vi "Normalize.vi"(8 "error in (no error)":errorcluster, 9 "Params":dbl[](array[numeric]), 10 "NISTData.NIDataArray":T3 {"Time Stamp" format="%^<%.3X\n%x>T"}, 11 "TVEMePe":dbl[][](array[numeric])) -> (0 "error out":errorcluster, 1 "Residual Histogram":T1(array[cluster]), 2 "MeanStdevSlopeSineAmpl":dbl[][](array[numeric]), 3 "Plot Out":cluster{dbl, "Time":dbl, dbl[][]}[](array[cluster]))   [LabVIEW 2014]
uses:
  typedefs/NIDataArray.ctl
  typedefs/NIData.ctl
  typedefs/PhasorRectangular.ctl
  <vilib>/Analysis/6fits.llb/Curve Fitting Criteria.ctl
  <vilib>/measure/matone.llb/Extract Single Tone Information 1 Chan.vi
  <vilib>/Analysis/NI_AALPro.lvlib
  <vilib>/Analysis/NI_AALBase.lvlib
  <vilib>/measure/NI_MAPro.lvlib
panel:
  out "Residual Error Distribution":T2(graph)
  out "Waveform Graph":cluster{dbl, "Time":dbl, dbl[][]}(graph)
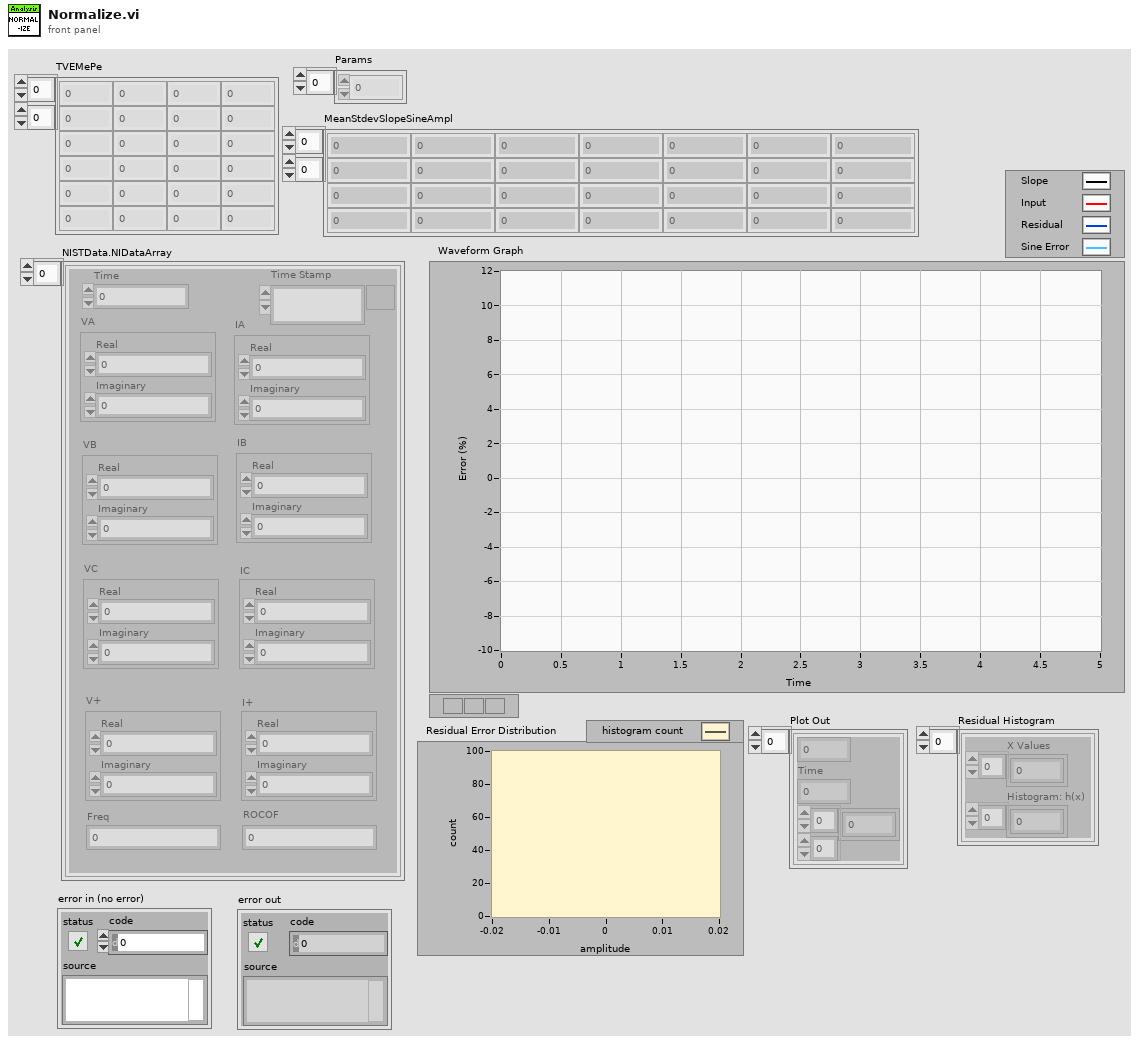
[diagram p1: front panel]
types:
  T1 = cluster{"X Values":dbl[], "Histogram: h(x)":i32[]}[]
  T2 = cluster{"X Values":dbl[], "Histogram: h(x)":i32[]}
  T3 = typedef "NIDataArray.ctl" = T4[]
  T4 = typedef "NIData.ctl" = cluster{"Time":dbl, "VA":T5, "VB":T5, "VC":T5, "V+":T5, "IA":T5, "IB":T5, "IC":T5, "I+":T5, "Freq":dbl, "ROCOF":dbl, "Time Stamp":timestamp}
  T5 = typedef "PhasorRectangular.ctl" = cluster{"Real":dbl, "Imaginary":dbl}
  T6 = enum32{"none", "input signal", "detected signal", "residual signal"}
  T7 = typedef "NI_AALPro.lvlib/Curve Fitting Criteria.ctl" = u16
  T8 = cluster{"exported time signal":waveform(dbl), "exported spectrum (dB)":cluster{"f0":dbl, "df":dbl, "dB Spectrum (Hann)":dbl[]}}
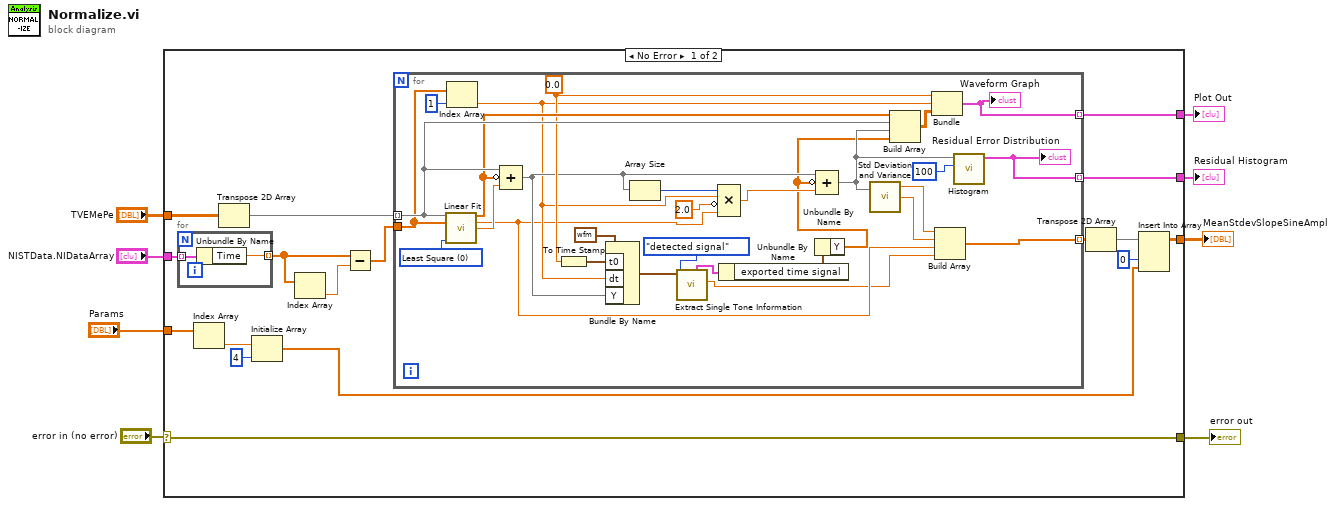
[diagram p0: block diagram]
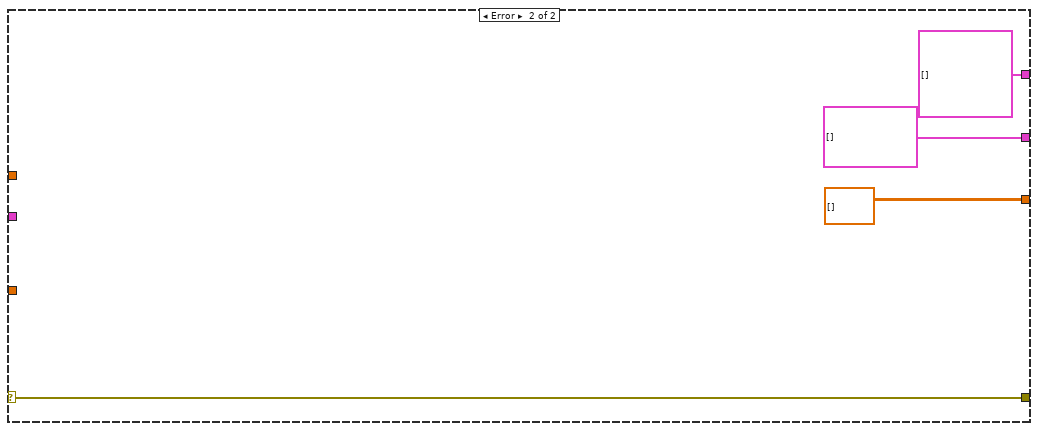
[diagram p2: hidden frame]
diagram:
  n1 = case shown="No Error" "error in (no error)" {
    selector: "error in (no error)" -> [w22 w60]
    tunnel: "NISTData.NIDataArray" -> [w25 _]
    tunnel: "TVEMePe" -> [w24 _]
    tunnel: [w13 dbl[][] []] -> w4
    tunnel: [w22 w60] -> w5
    tunnel: "Params" -> [w16 _]
    tunnel: [w10 cluster{dbl, "Time":dbl, dbl[][]}[] []] -> w2
    tunnel: [w9 T1 []] -> w1
    frame No Error {
      n2 = for {
        tunnel: w25 -> [w56] mode=indexing
        tunnel: [w55] -> w20 mode=indexing
        n3 = Unbundle By Name(w56) -> ("Time"=w55:dbl)
      }
      n4 = Index Array(array=w16) -> (element=w15:dbl)  [unwired: 1 in]
      n5 = Transpose 2D Array(2D array=w24) -> (transposed array=w21:dbl[][])
      n6 = Initialize Array(w15, 4 ("dimension size")) -> (w11:dbl[])
      n7 = Index Array(array=w20) -> (element=w19:dbl)  [unwired: 1 in]
      n8 = Subtract(x=w20, y=w19) -> (x-y=w18:dbl[])
      n9 = for {
        tunnel: w21 -> [w53] mode=indexing
        tunnel: w18 -> [w45]
        tunnel: [w51] -> w23 mode=indexing
        tunnel: [w27] -> w10 mode=indexing
        tunnel: [w26] -> w9 mode=indexing
        w42 = 0.0
        w54 = T7 0 items=["Least Square", "Least Absolute Residual", "Bisquare"] ("method")
        n10 = call <vilib>:"Linear Fit.vi"("Y"=w53, "X"=w45, "method"=w54) -> ("Best Linear Fit"=w52:dbl[], "slope"=w30:dbl, "intercept"=w36:dbl)  [unwired: 8 in, 2 out]
        n11 = Index Array(array=w45, index=1) -> (element=w33:dbl)
        n12 = Compound Arithmetic op=ADD(w53, invert w52, w36) -> (w35:dbl[])
        n13 = To Time Stamp(1:w42) -> (0:w43:timestamp)
        n14 = Bundle By Name(cluster=waveform(dbl) {"t0"=timestamp(0 s since 1904-01-01), "dt"=1.0, "Y"=[]} ("time signal in"), "t0"=w43, "dt"=w33, "Y"=w35) -> (w41:waveform(dbl))
        n15 = Array Size(array=w35) -> (size(s)=w34:i32)
        n16 = call-poly <vilib>:"Extract Single Tone Information.vi"("export mode"=T6."detected signal", "time signal in"=w41) -> ("detected amplitude"=w28:dbl, "exported signals"=w38:T8)  [unwired: 4 in, 4 out]
        n17 = Compound Arithmetic op=MULTIPLY(w34, w33, invert 2.0 ("value"), w30) -> (w31:dbl)
        n18 = Unbundle By Name(w38) -> ("exported time signal"=w37:waveform(dbl))
        n19 = Unbundle By Name(w37) -> ("Y"=w29:dbl[])
        n20 = Compound Arithmetic op=ADD(w35, invert w29, w31) -> (w40:dbl[])
        n21 = call <vilib>:"Std Deviation and Variance.vi"("X"=w40) -> ("mean"=w47:dbl, "standard deviation"=w48:dbl)  [unwired: 1 in, 1 out]
        n22 = Build Array(w52, w53, w40, w29) -> (w50:dbl[][])
        n23 = Bundle(w42, "Time"=w33, w50) -> (w27:cluster{dbl, "Time":dbl, dbl[][]})  [unwired: 1 in]
        "Waveform Graph" <- w27
        n24 = Build Array(w47, w48, w30, w28) -> (w51:dbl[])
        n25 = call <vilib>:"Histogram.vi"("intervals"=100, "X"=w40) -> ("Histogram Graph"=w26:T2)  [unwired: 6 in, 3 out]
        "Residual Error Distribution" <- w26
      }
      n26 = Transpose 2D Array(2D array=w23) -> (transposed array=w17:dbl[][])
      n27 = Insert Into Array(array=w17, index (col)=0 ("disabled index (col)"), new element=w11) -> (w13:dbl[][])  [unwired: 1 in]
    }
    frame Error {
    }
  }
  "error out" <- w5
  "MeanStdevSlopeSineAmpl" <- w4
  "Plot Out" <- w2
  "Residual Histogram" <- w1
